vi "Delegate & Prioritize.vi"(8 "error in (no error)":errorcluster) -> (0 "error out":errorcluster)   [LabVIEW 2015, in "Sprocket.lvlib"]
uses:
  lib/Sprocket.lvlib
  Refname/Queues.ctl
  Refname/Refname to String (Queue).vi
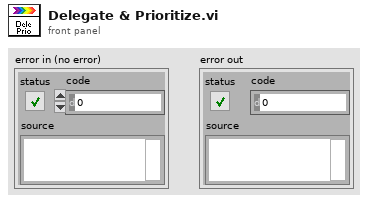
[diagram p1: front panel]
types:
  T1 = typedef "Sprocket.lvlib/Queues.ctl" = enum16{"Input", "Drive", "Collector", "Shifter", "Wedge"}
  T2 = typedef "Sprocket.lvlib/Action.ctl" = cluster{"Name":T3, "Priority":i32, "Data":variant}
  T3 = typedef "Sprocket.lvlib/Action Name.ctl" = enum16{"No Action", "Drive Train Left", "Drive Train Right", "Drive Train Both", "Collector Motor Roll", "Collector Motor Eject", "Collector Motor Collect", "Collector Motor Stop", "Collector Extend", "Collector Retract", "Shifter High", "Shifter Low", "Collector Motor Stall"}
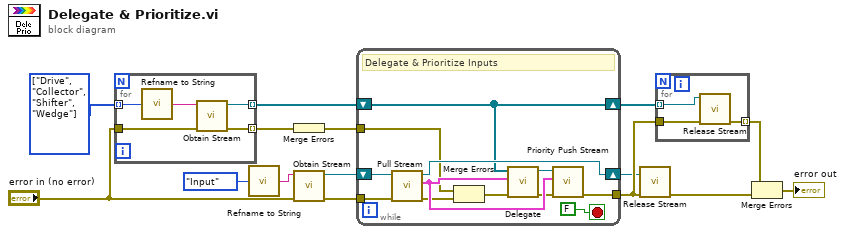
[diagram p0: block diagram]
diagram:
  w5 = T1[] [enum."Drive", enum."Collector", enum."Shifter", enum."Wedge"] items=["Input", "Drive", "Collector", "Shifter", "Wedge"]
  n1 = for {
    tunnel: w5 -> [w19] mode=indexing
    tunnel: [w18] -> w1 mode=indexing
    tunnel: "error in (no error)" -> [w17]
    tunnel: [w16] -> w3 mode=indexing
    n2 = call-poly "Refname to String.vi"("Queue Refname"=w19) -> ("Refnum Name"=w20:string)
    n3 = call "Obtain Stream.vi"("error in (no error)"=w17, "Name"=w20) -> ("error out"=w16:errorcluster, "stream out"=w18:refnum<queue>)  [unwired: 8 in]
  }
  n4 = call-poly "Refname to String.vi"("Queue Refname"=Queues."Input" ("Refname (Queue)")) -> ("Refnum Name"=w14:string)
  n5 = Merge Errors(w3) -> (w2:errorcluster)
  n6 = call "Obtain Stream.vi"("error in (no error)"="error in (no error)", "Name"=w14) -> ("error out"=w10:errorcluster, "stream out"=w9:refnum<queue>)  [unwired: 8 in]
  n7 = while {
    tunnel: w10 -> [w32]
    shift-right: [w30] -> w11
    shift-left: w9 -> [w31]
    shift-right: [w29] -> w12
    shift-left: w1 -> [w29]
    tunnel: [w25] -> w13
    tunnel: w2 -> [w21]
    stop <- FALSE stop-if-true
    # "Delegate & Prioritize Inputs"
    n8 = call "Pull Stream.vi"("error in (no error)"=w32, "stream in"=w31) -> ("error out"=w22:errorcluster, "element"=w27:T2, "queue out"=w30:refnum<queue>)  [unwired: 6 in, 1 out]
    n9 = Merge Errors(w21, w22) -> (w23:errorcluster)
    n10 = call "Delegate.vi"("error in (no error)"=w23, "Action"=w27, "Subsystems"=w29) -> ("error out"=w26:errorcluster, "Delegate"=w28:refnum<queue>)  [unwired: 7 in]
    n11 = call "Priority Push Stream.vi"("error in (no error)"=w26, "Action"=w27, "Subsystem in"=w28) -> ("error out"=w25:errorcluster)  [unwired: 7 in, 1 out]
  }
  n12 = call "Release Stream.vi"("error in (no error)"=w13, "stream in"=w11) -> ("error out"=w7:errorcluster)  [unwired: 8 in, 1 out]
  n13 = for {
    tunnel: w12 -> [w35] mode=indexing
    tunnel: w13 -> [w34]
    tunnel: [w33] -> w8 mode=indexing
    n14 = call "Release Stream.vi"("error in (no error)"=w34, "stream in"=w35) -> ("error out"=w33:errorcluster)  [unwired: 8 in, 1 out]
  }
  n15 = Merge Errors(w8, w7) -> (→"error out":errorcluster)
